vi "BallPlacementEnemyRole.vi"(9 "Game in":refnum<class "Game.lvclass">, 10 "Robot in":refnum<class "Robot.lvclass">, 11 "BallPlacementEnemyRole in":refnum<class "BallPlacementEnemyRole.lvclass">) -> (0 "tactic index out":i32, 1 "Game out":refnum<class "Game.lvclass">, 2 "Robot out":refnum<class "Robot.lvclass">, 3 "BallPlacementEnemyRole out":refnum<class "BallPlacementEnemyRole.lvclass">)   [LabVIEW 2020, in "BallPlacementEnemyRole.lvclass"]
uses:
  BallPlacementEnemyRole.lvclass
  C:/RoboIME/SSL_AI/Role_class/Role.lvclass
  Robot_class/Robot.lvclass
  Game_class/Game.lvclass
  Role_class/Role.lvclass/Role.ctl
  Role_class/Read Tacticbook.vi
  Role_class/Read tactic_index.vi
  Role_class/Write Tacticbook.vi
  Role_class/Write tactic_index.vi
  Tacticbook_class/Tacticbook.lvclass
  BallPlacementEnemyTactic_class/BallPlacementEnemyTactic.lvclass
panel:
  out "error out":errorcluster
  in  "error in (no error)":errorcluster
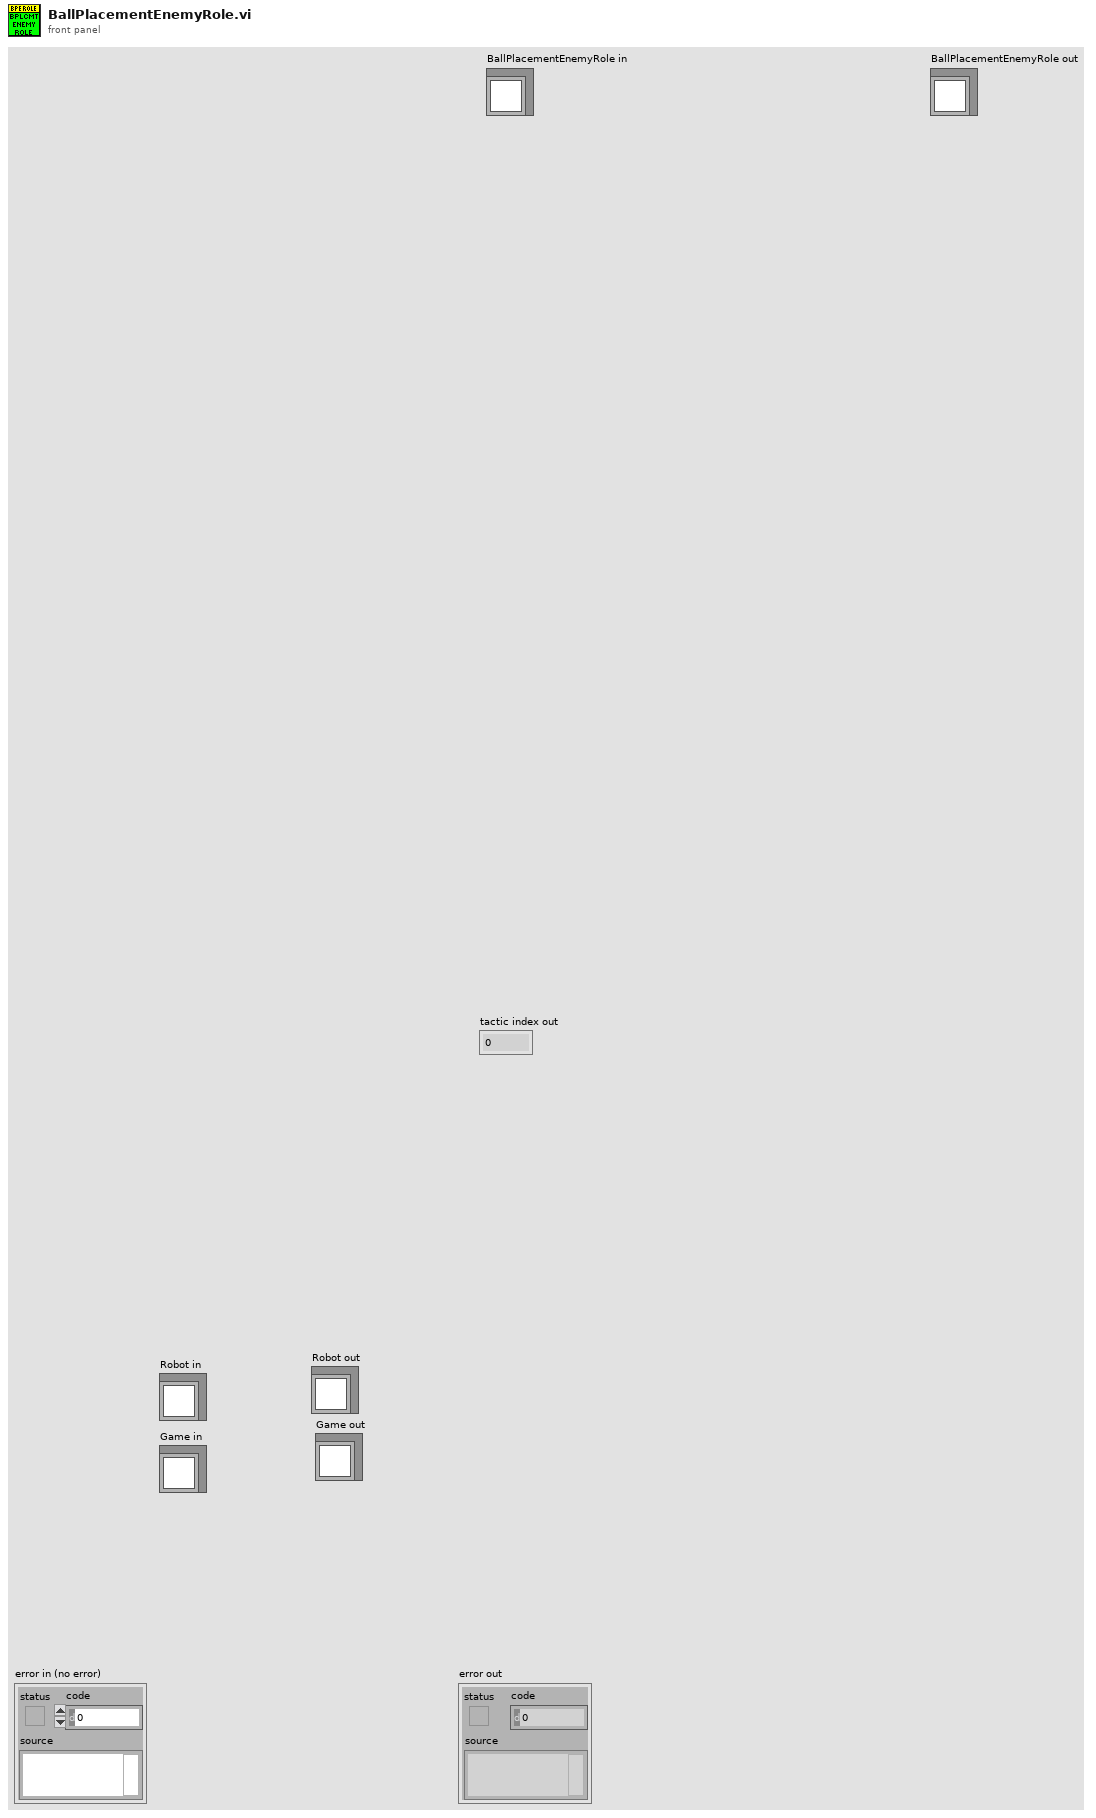
[diagram p1: front panel]
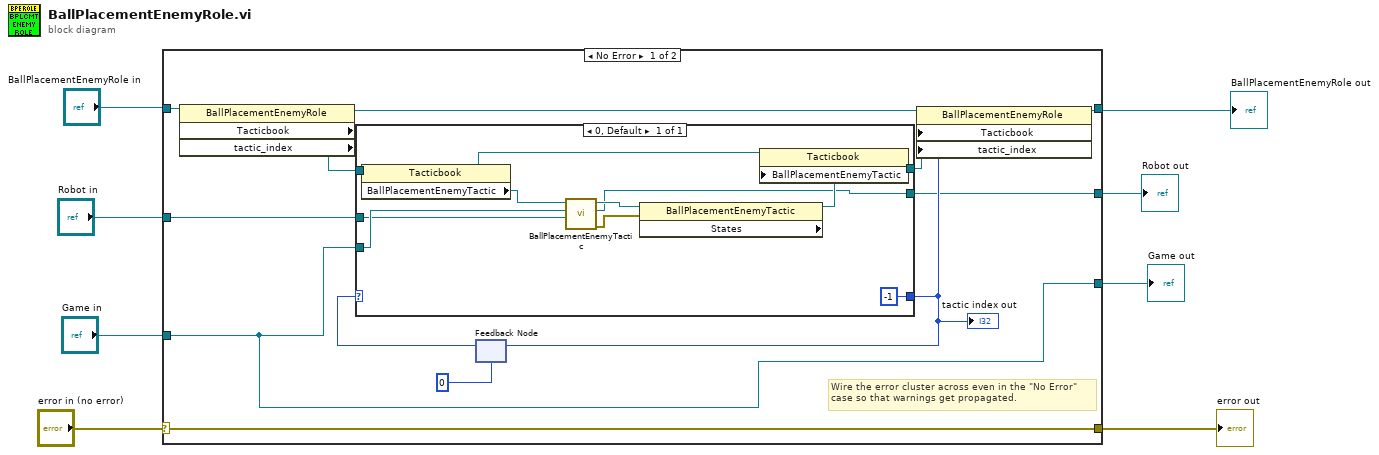
[diagram p0: block diagram]
diagram:
  n1 = case shown="No Error" "error in (no error)" {
    selector: "error in (no error)" -> [w20 w35]
    tunnel: [w20 w35] -> w7
    tunnel: [w18 w34] -> w3
    tunnel: "BallPlacementEnemyRole in" -> [w19 w34]
    tunnel: "Robot in" -> [w12 w33]
    tunnel: [w11 w33] -> w6
    tunnel: [w9 w32] -> w5
    tunnel: "Game in" -> [w9 w32]
    frame No Error {
      # "Wire the error cluster across even in the \"No Error\"\ncase so that warnings get propagated."
      n2 = property class="BallPlacementEnemyRole" props=["Tacticbook", "tactic_index"](reference=w19) -> (reference out=w17:refnum<class "BallPlacementEnemyRole.lvclass">, "Tacticbook"=w14:refnum<class "Tacticbook.lvclass">)  [unwired: 1 in, 2 out]
      n3 = feedback #1(0) -> (w15:i32)
      n4 = case shown="0, Default" w15 {
        tunnel: [-1] -> w13
        tunnel: w14 -> [w31]
        tunnel: w12 -> [w24]
        tunnel: [w22] -> w11
        tunnel: [w28] -> w10
        tunnel: w9 -> [w25]
        frame 0, Default {
          n5 = property class="Tacticbook"(reference=w31) -> (reference out=w30:refnum<class "Tacticbook.lvclass">, "BallPlacementEnemyTactic"=w26:refnum<class "BallPlacementEnemyTactic.lvclass">)  [unwired: 1 in, 1 out]
          n6 = call "BallPlacementEnemyTactic.vi"("Robot"=w24, "Game"=w25, "BallPlacementEnemyTactic in"=w26) -> ("error out"=w21:errorcluster, "Robot out"=w22:refnum<class "Robot.lvclass">, "BallPlacementEnemyTactic out"=w23:refnum<class "BallPlacementEnemyTactic.lvclass">)  [unwired: 6 in]
          n7 = property class="BallPlacementEnemyTactic" props=["States"](reference=w23, error in=w21) -> (reference out=w29:refnum<class "BallPlacementEnemyTactic.lvclass">)  [unwired: 2 out]
          n8 = property class="Tacticbook"(reference=w30, "BallPlacementEnemyTactic"=w29) -> (reference out=w28:refnum<class "Tacticbook.lvclass">)  [unwired: 1 in, 1 out]
        }
      }
      "tactic index out" <- w13
      n9 = feedback-in #1(w13) -> ()
      n10 = property class="BallPlacementEnemyRole"(reference=w17, "Tacticbook"=w10, "tactic_index"=w13) -> (reference out=w18:refnum<class "BallPlacementEnemyRole.lvclass">)  [unwired: 1 in, 1 out]
    }
    frame Error {
    }
  }
  "BallPlacementEnemyRole out" <- w3
  "error out" <- w7
  "Robot out" <- w6
  "Game out" <- w5
